vi "dfd_Raised Cosine Filter Coefficients.vi"(5 "type":enum16{"Raised Cosine", "Root Raised Cosine"}(ring), 7 "#band":i32, 8 "error in (no error)":errorcluster, 10 "roll off":dbl=0.1 format="%.2f", 11 "order":i32=2) -> (0 "error out":errorcluster, 3 "coefficients b":dbl[](array[numeric]) format="%.2f")   [LabVIEW 2017, in "NI_DigFilter_Process.lvlib"]
uses:
  <vilib>/addons/Digital Filter Design/NI_DigFilter_Process.lvlib
  <vilib>/Analysis/1siggen.llb/Ramp Pattern by Samples.vi
  <vilib>/Analysis/NI_AALBase.lvlib
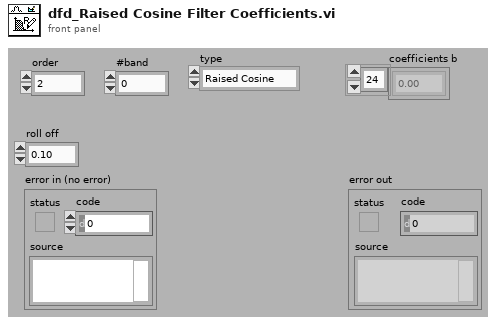
[diagram p1: front panel]
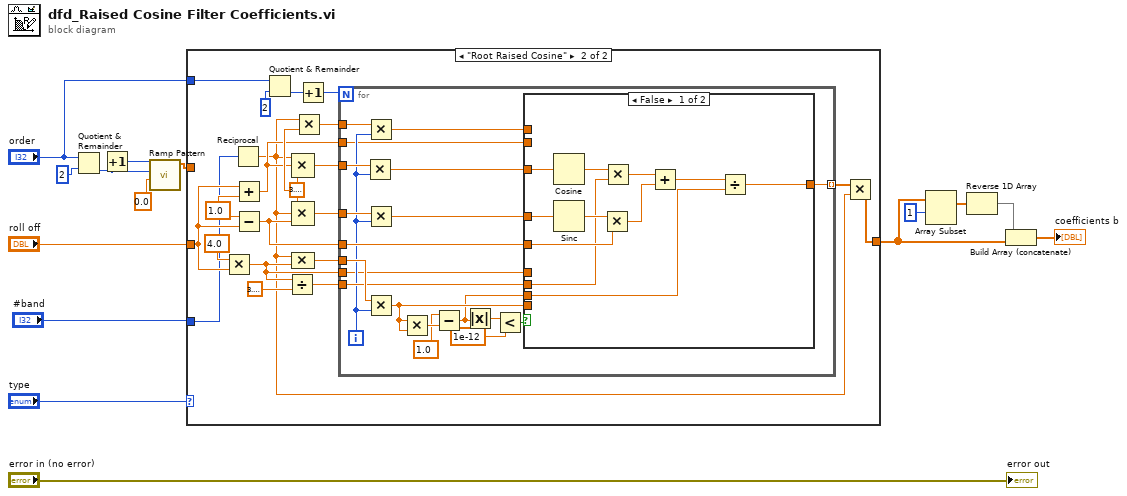
[diagram p0: block diagram]
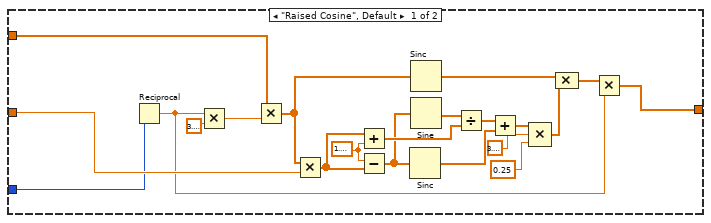
[diagram p2: hidden frame]
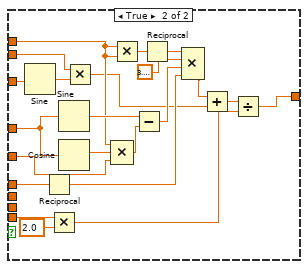
[diagram p3: hidden frame]
diagram:
  n1 = Quotient & Remainder(x="order", y=2) -> (floor(x/y)=w9:i32)  [unwired: 1 out]
  n2 = Increment(x=w9) -> (x+1=w12:i32)
  n3 = call-poly <vilib>:"Ramp Pattern.vi"("start"=0.0, "end"=w9, "samples"=w12) -> ("Ramp Pattern"=w8:dbl[])  [unwired: 7 in, 1 out]
  n4 = case shown="\"Root Raised Cosine\"" "type" {
    tunnel: w8 -> [w20 _]
    tunnel: "roll off" -> [w21 w41]
    tunnel: "#band" -> [w18 w40]
    tunnel: [w16 w38] -> w5
    tunnel: "order" -> [_ w39]
    frame "Raised Cosine", Default {
      w34 = 1.5707963267948966
      n5 = Reciprocal(x=w18) -> (1/x=w17:dbl)
      n6 = Multiply(x=w17, y=3.141592653589793) -> (x*y=w25:dbl)
      n7 = Multiply(x=w20, y=w25) -> (x*y=w24:dbl[])
      n8 = Multiply(x=w24, y=w21) -> (x*y=w26:dbl[])
      n9 = Add(x=w26, y=w34) -> (x+y=w23:dbl[])
      n10 = Subtract(x=w34, y=w26) -> (x-y=w22:dbl[])
      n11 = Sinc(1:w22) -> (0:w31:dbl[])
      n12 = Sinc(1:w24) -> (0:w35:dbl[])
      n13 = Sine(x=w22) -> (sin(x)=w33:dbl[])
      n14 = Divide(x=w33, y=w23) -> (x/y=w32:dbl[])
      n15 = Add(x=w32, y=w31) -> (x+y=w30:dbl[])
      n16 = Compound Arithmetic op=MULTIPLY(w30, 3.141592653589793, 0.25) -> (w29:dbl[])
      n17 = Compound Arithmetic op=MULTIPLY(w35, w29) -> (w19:dbl[])
      n18 = Multiply(x=w19, y=w17) -> (x*y=w16:dbl[])
    }
    frame "Root Raised Cosine" {
      w53 = 3.141592653589793
      w54 = 1.0 ("y")
      n19 = Multiply(x=4.0 ("Input"), y=w41) -> (x*y=w43:dbl)
      n20 = Reciprocal(x=w40) -> (1/x=w37:dbl)
      n21 = Add(x=w41, y=w54) -> (x+y=w42:dbl)
      n22 = Subtract(x=w54, y=w41) -> (x-y=w48:dbl)
      n23 = Quotient & Remainder(x=w39, y=2) -> (floor(x/y)=w55:i32)  [unwired: 1 out]
      n24 = Divide(x=w43, y=3.141592653589793) -> (x/y=w46:dbl)
      n25 = Compound Arithmetic op=MULTIPLY(w37, w42, w53) -> (w52:dbl)
      n26 = Compound Arithmetic op=MULTIPLY(w53, w37, w48) -> (w51:dbl)
      n27 = Compound Arithmetic op=MULTIPLY(w37, w43) -> (w50:dbl)
      n28 = Multiply(x=w37, y=w53) -> (x*y=w44:dbl)
      n29 = Increment(x=w55) -> (x+1=w56:i32)
      n30 = for {
        N: w56 -> [_]
        tunnel: w52 -> [w75]
        tunnel: w51 -> [w76]
        tunnel: w50 -> [w77]
        tunnel: w48 -> [w70]
        tunnel: w46 -> [w69]
        tunnel: [w68] -> w45 mode=indexing
        tunnel: w44 -> [w67]
        tunnel: w43 -> [w64]
        tunnel: w42 -> [w63]
        i -> [w66]
        n31 = Multiply(x=w75, y=w66) -> (x*y=w74:dbl)
        n32 = Multiply(x=w67, y=w66) -> (x*y=w65:dbl)
        n33 = Multiply(x=w76, y=w66) -> (x*y=w73:dbl)
        n34 = Multiply(x=w77, y=w66) -> (x*y=w62:dbl)
        n35 = Multiply(x=w62, y=w62) -> (x*y=w72:dbl)
        n36 = Subtract(x=1.0 ("y"), y=w72) -> (x-y=w58:dbl)
        n37 = Absolute Value(x=w58) -> (abs(x)=w61:dbl)
        n38 = Less?(x=w61, y=1e-12) -> (x < y?=w59:bool)
        n39 = case shown="False" w59 {
          tunnel: w74 -> [w88 w99]
          tunnel: w73 -> [w87 w110]
          tunnel: w70 -> [w85 w89]
          tunnel: w69 -> [w83 _]
          tunnel: w58 -> [w79 _]
          tunnel: [w78 w90] -> w68
          tunnel: w65 -> [_ w106]
          tunnel: w64 -> [_ w102]
          tunnel: w63 -> [_ w97]
          tunnel: w62 -> [_ w93]
          frame False {
            n40 = Cosine(x=w88) -> (cos(x)=w84:dbl)
            n41 = Sinc(1:w87) -> (0:w86:dbl)
            n42 = Multiply(x=w86, y=w85) -> (x*y=w81:dbl)
            n43 = Multiply(x=w84, y=w83) -> (x*y=w82:dbl)
            n44 = Add(x=w82, y=w81) -> (x+y=w80:dbl)
            n45 = Divide(x=w80, y=w79) -> (x/y=w78:dbl)
          }
          frame True {
            n46 = Sine(x=w99) -> (sin(x)=w98:dbl)
            n47 = Reciprocal(x=w102) -> (1/x=w101:dbl)
            n48 = Multiply(x=w93, y=2.0) -> (x*y=w91:dbl)
            n49 = Sine(x=w110) -> (sin(x)=w109:dbl)
            n50 = Cosine(x=w110) -> (cos(x)=w107:dbl)
            n51 = Multiply(x=w97, y=w98) -> (x*y=w95:dbl)
            n52 = Compound Arithmetic op=MULTIPLY(w106, w107, w89) -> (w108:dbl)
            n53 = Multiply(x=w106, y=w106) -> (x*y=w105:dbl)
            n54 = Subtract(x=w109, y=w108) -> (x-y=w100:dbl)
            n55 = Reciprocal(x=w105) -> (1/x=w104:dbl)
            n56 = Compound Arithmetic op=MULTIPLY(w104, 3.141592653589793, w100, w101) -> (w96:dbl)
            n57 = Add(x=w96, y=w95) -> (x+y=w94:dbl)
            n58 = Divide(x=w94, y=w91) -> (x/y=w90:dbl)
          }
        }
      }
      n59 = Multiply(x=w45, y=w37) -> (x*y=w38:dbl[])
    }
  }
  n60 = Array Subset(array=w5, index=1) -> (w6:dbl[])  [unwired: 1 in]
  n61 = Reverse 1D Array(array=w6) -> (reversed array=w4:dbl[])
  n62 = Build Array (concatenate)(w4, w5) -> (→"coefficients b":dbl[])
  "error out" <- "error in (no error)"
